vi "fgv_ekf_motion-model.vi"(10 "u":T1, 11 "x_true":T1) -> (3 "x_true out":T1)   [LabVIEW 2019]
uses:
  <vilib>/Analysis/Matrix/Datatypes/RealMatrix.ctl
  Ctrl/cmd_common.ctl
  <vilib>/Analysis/baseanly.llb/Real A x B.vi
  <vilib>/Analysis/Matrix/Numeric/Add/Add - RM,RM.vi
  <vilib>/Analysis/Matrix/NI_Matrix.lvlib
  <vilib>/Analysis/NI_AALBase.lvlib
panel:
  out "열 x_true":i32
  out "행 x_true":i32
  out "B":T1
  out "행 F":i32
  out "열 F":i32
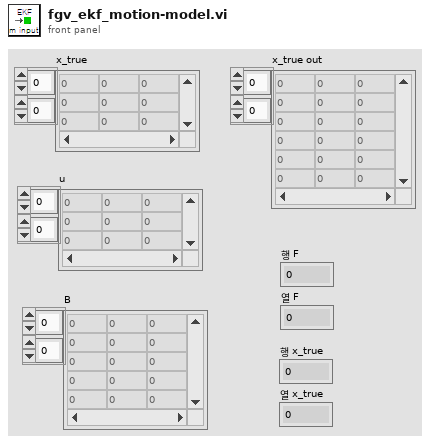
[diagram p1: front panel]
types:
  T1 = typedef "NI_Matrix.lvlib/RealMatrix.ctl" = dbl[][]
  T2 = typedef "cmd_common.ctl" = enum16{"read", "write"}
  T3 = cluster{"Q":T1, "R":T1, "input Noise":T1, "GPS noise":T1, "DT":dbl}
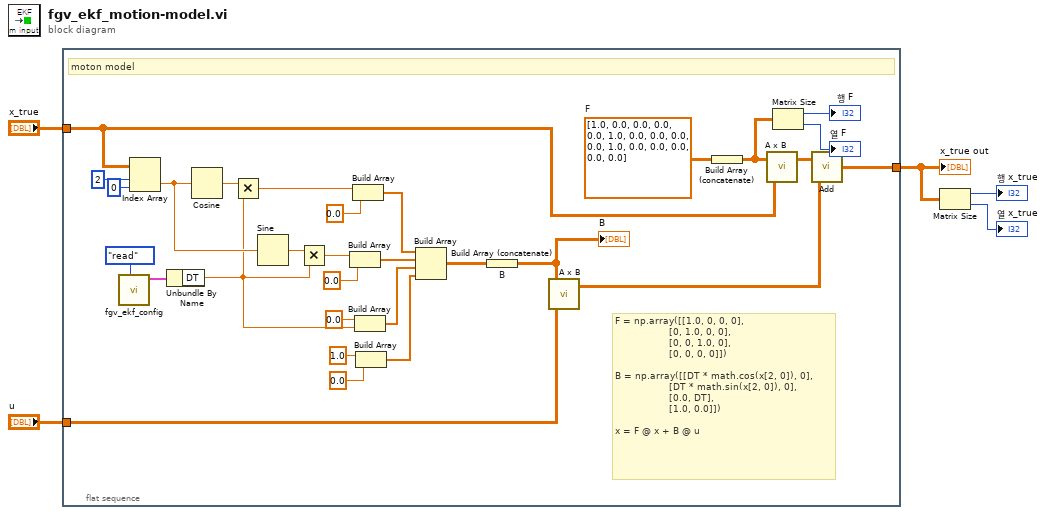
[diagram p0: block diagram]
diagram:
  n1 = flat-sequence {
    tunnel: "x_true" -> [w9]
    tunnel: "u" -> [w8]
    tunnel: [w13] -> w1
    frame #0 {
      w16 = dbl[][] [[1.0, 0.0, 0.0, 0.0], [0.0, 1.0, 0.0, 0.0], [0.0, 0.0, 1.0, 0.0], [0.0, 0.0, 0.0, 0.0]]  # F
      # "F = np.array([[1.0, 0, 0, 0],\n                  [0, 1.0, 0, 0],\n                  [0, 0, 1.0, 0],\n                  [0, 0, 0, 0]])\n\nB = np.array([[DT * math.cos(x[2, 0]), 0],\n                  [DT * math.sin(x[2, 0]), 0],\n                  [0.0, DT],\n                  [1.0, 0.0]])\n\nx = F @ x + B @ u"
      # "moton model"
      n2 = call "fgv_ekf_config.vi"("cmd"=cmd_common."read") -> ("set var out"=w7:T3)  [unwired: 10 in]
      n3 = Index Array(array=w9, index (row)=2 ("인덱스 (행)"), index (col)=0 ("인덱스 (열)")) -> (element=w31:dbl)
      n4 = Unbundle By Name(w7) -> ("DT"=w6:dbl)
      n5 = Cosine(x=w31) -> (cos(x)=w33:dbl)
      n6 = Multiply(x=w33, y=w6) -> (x*y=w30:dbl)
      n7 = Sine(x=w31) -> (sin(x)=w32:dbl)
      n8 = Multiply(x=w32, y=w6) -> (x*y=w27:dbl)
      n9 = Build Array(w27, 0.0 ("원소")) -> (w21:dbl[])
      n10 = Build Array(w30, 0.0 ("원소")) -> (w20:dbl[])
      n11 = Build Array(0.0 ("원소"), w6) -> (w22:dbl[])
      n12 = Build Array(1.0 ("원소"), 0.0 ("원소")) -> (w23:dbl[])
      n13 = Build Array(w20, w21, w22, w23) -> (w19:dbl[][])
      n14 = Build Array (concatenate) "B"(w19) -> (w18:T1)
      "B" <- w18
      n15 = call-poly <vilib>:"A x B.vi"("B"=w8, "A"=w18) -> ("A x B"=w17:T1)  [unwired: 1 out]
      n16 = Build Array (concatenate)(w16) -> (w12:T1)
      n17 = call-poly <vilib>:"A x B.vi"("B"=w9, "A"=w12) -> ("A x B"=w15:T1)  [unwired: 1 out]
      n18 = Matrix Size(0:w12) -> (1:→"행 F":i32, 2:→"열 F":i32)
      n19 = call-poly <vilib>:"Add.vi"("Real Matrix B"=w17, "Real Matrix A"=w15) -> ("A + B"=w13:T1)
    }
  }
  n20 = Matrix Size(0:w1) -> (1:→"행 x_true":i32, 2:→"열 x_true":i32)
  "x_true out" <- w1
